vi "Copy .LLB to NI VeriStand dir.vi"(5 "Files Generated by Build":path[](array[path]), 6 "Top Level/Always Included VIs":path[](array[path]), 7 "Destination Path":path, 8 "error in (no error)":errorcluster, 9 "Target Name":string, 10 "Build Specification Name":string, 11 "Project Path":path) -> (0 "error out":errorcluster)   [LabVIEW 2026]
doc: "This VI is called after each run of a build specification. The VI will copy the generated LLB (Engine or System Explorer) into the VeriStand Custom Device folder (...\\Documents\\National Instruments\\NI VeriStand 2013...)."
uses:
  <vilib>/Utility/sysdir.llb/System Directory Type.ctl
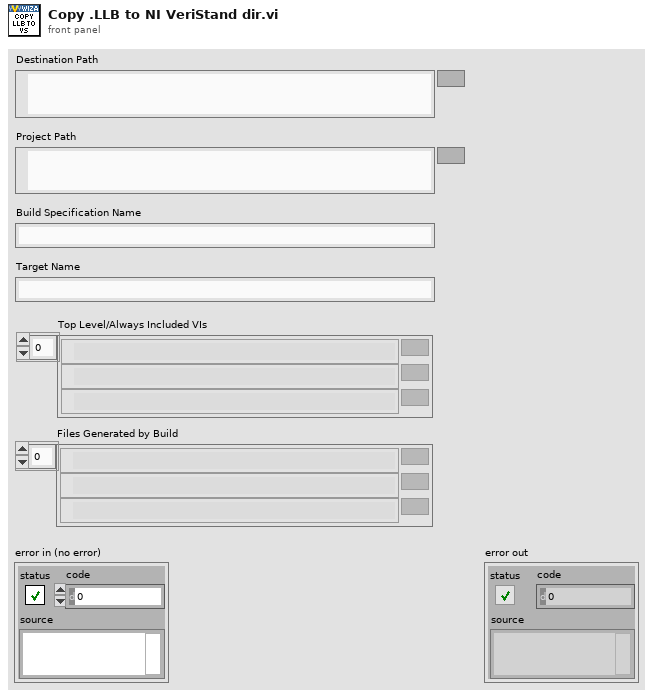
[diagram p1: front panel]
types:
  T1 = typedef "System Directory Type.ctl" = i32
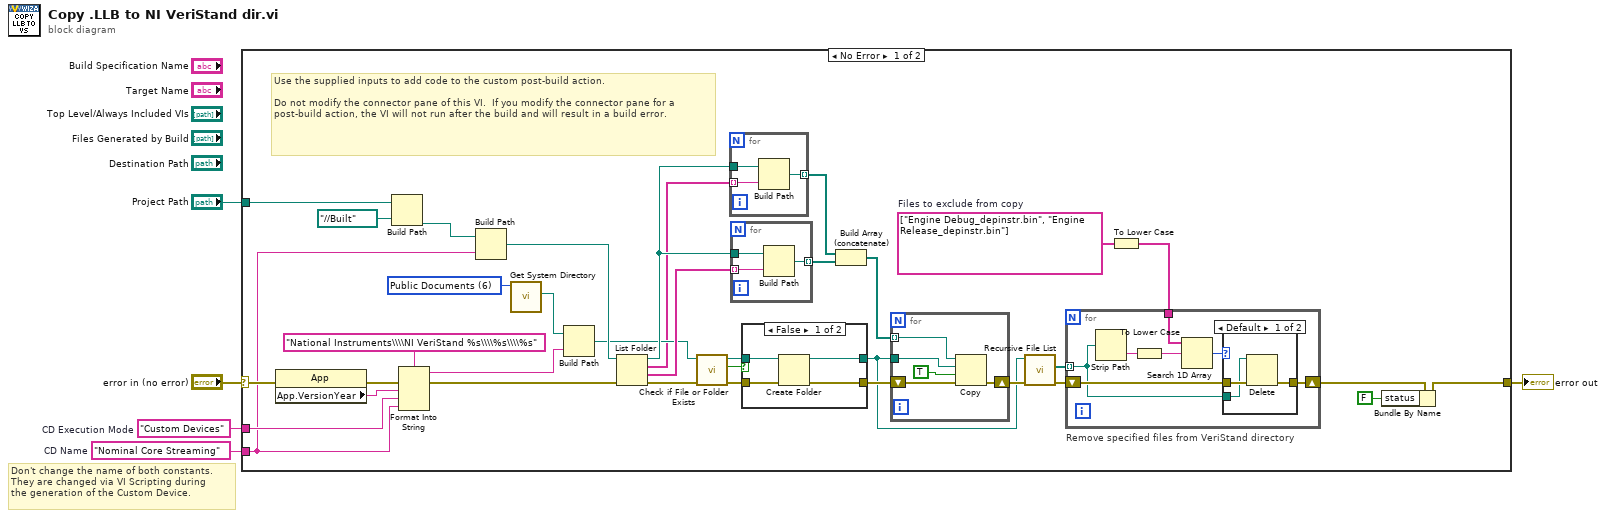
[diagram p0: block diagram]
diagram:
  w2 = "Nominal Core Streaming"  # CD Name
  w3 = "Custom Devices"  # CD Execution Mode
  # "Don't change the name of both constants.\nThey are changed via VI Scripting during\nthe generation of the Custom Device."
  n1 = case shown="No Error" "error in (no error)" {
    selector: "error in (no error)" -> [w21 w69]
    tunnel: [w7 w69] -> w1
    tunnel: "Project Path" -> [w17 _]
    tunnel: w3 -> [w22 _]
    tunnel: w2 -> [w19 _]
    frame No Error {
      w14 = string[] ["Engine Debug_depinstr.bin", "Engine Release_depinstr.bin"]  # Files to exclude from copy
      w27 = T1 6 items=["User Home"=0, "User Desktop"=1, "User Documents"=2, "User Application Data"=3, "User Preferences"=4, "User Temporary"=5, "Public Documents"=6, "Public Application Data"=7, "Public Preferences"=8, "Public Cache"=13, "System Core Libraries"=9, "System Installed Libraries"=10, "Application Files"=11, "Boot Volume Root"=12] ("system directory type")
      # "Use the supplied inputs to add code to the custom post-build action.\n\nDo not modify the connector pane of this VI.  If you modify the connector pane for a post-build action, the VI will not run after the build and will result in a build error."
      n2 = property class="App"(error in=w21) -> (error out=w26:errorcluster, "App.VersionYear"=w25:string)  [unwired: 1 in, 1 out]
      n3 = Build Path(base path=w17, name or relative path=path "../../Built") -> (appended path=w30:path)
      n4 = Format Into String(format string="National Instruments\\\\NI VeriStand %s\\\\%s\\\\%s" ("name or relative path"), error in=w26, w25, w22, w19) -> (resulting string=w29:string, error out=w20:errorcluster)  [unwired: 1 in]
      n5 = Build Path(base path=w30, name or relative path=w19) -> (appended path=w32:path)
      n6 = call <vilib>:"Get System Directory.vi"("system directory type"=w27) -> ("system directory"=w28:path)  [unwired: 10 in]
      n7 = Build Path(base path=w28, name or relative path=w29) -> (appended path=w23:path)
      n8 = List Folder(path=w32, error in=w20) -> (path out=w34:path, filenames=w15:string[], folder names=w35:string[], error out=w31:errorcluster)  [unwired: 2 in]
      n9 = call <vilib>:"Check if File or Folder Exists.vi"("error in (no error)"=w31, "path"=w23) -> ("error out"=w36:errorcluster, "file or folder exists?"=w38:bool, "dup path"=w37:path)  [unwired: 7 in]
      n10 = for {
        tunnel: w15 -> [w67] mode=indexing
        tunnel: w34 -> [w68]
        tunnel: [w66] -> w40 mode=indexing
        n11 = Build Path(base path=w68, name or relative path=w67) -> (appended path=w66:path)
      }
      n12 = for {
        tunnel: w35 -> [w64] mode=indexing
        tunnel: w34 -> [w65]
        tunnel: [w63] -> w33 mode=indexing
        n13 = Build Path(base path=w65, name or relative path=w64) -> (appended path=w63:path)
      }
      n14 = case shown="False" w38 {
        tunnel: w37 -> [w55 w57]
        tunnel: w36 -> [w54 w56]
        tunnel: [w53 w57] -> w9
        tunnel: [w52 w56] -> w16
        frame False {
          n15 = Create Folder(path (use dialog)=w55, error in=w54) -> (created path=w53:path, error out=w52:errorcluster)  [unwired: 1 in, 1 out]
        }
        frame True {
        }
      }
      n16 = Build Array (concatenate)(w40, w33) -> (w39:path[])
      n17 = for {
        tunnel: w39 -> [w59] mode=indexing
        shift-right: [w60] -> w10
        shift-left: w16 -> [w61]
        tunnel: w9 -> [w58]
        n18 = Copy(8:w61, 9:TRUE ("overwrite (F)"), 10:w58, 11:w59) -> (0:w60:errorcluster)  [unwired: 1 in, 2 out]
      }
      n19 = call <vilib>:"Recursive File List.vi"("error in (no error)"=w10, "Folder Path"=w9) -> ("error out"=w13:errorcluster, "All Files in Dir"=w12:path[])  [unwired: 5 in, 3 out]
      n20 = To Lower Case(string=w14) -> (all lower case string=w11:string[])
      n21 = for "Remove specified files from VeriStand directory" {
        shift-right: [w42] -> w8
        shift-left: w13 -> [w44]
        tunnel: w12 -> [w41] mode=indexing
        tunnel: w11 -> [w45]
        n22 = Strip Path(path=w41) -> (name=w47:string)  [unwired: 1 out]
        n23 = To Lower Case(string=w47) -> (all lower case string=w46:string)
        n24 = Search 1D Array(1D array=w45, element=w46) -> (index of element=w43:i32)  [unwired: 1 in]
        n25 = case shown="Default" w43 {
          tunnel: w44 -> [w50 w51]
          tunnel: [w49 w51] -> w42
          tunnel: w41 -> [w48 _]
          frame Default {
            n26 = Delete(path (use dialog)=w48, error in=w50) -> (error out=w49:errorcluster)  [unwired: 3 in, 2 out]
          }
          frame -1 {
          }
        }
      }
      n27 = Bundle By Name(cluster=w8, "status"=FALSE) -> (w7:errorcluster)
    }
    frame Error {
    }
  }
  "error out" <- w1
